vi "Set JSON Data.vi"(7 "VI Reference":refnum<vi>, 8 "error in (no error)":errorcluster, 10 "Value":string, 11 "String In":refnum<class "Cluster.lvclass">) -> (0 "error out":errorcluster, 3 "String Out":refnum<class "Cluster.lvclass">)   [LabVIEW 2017, in "Front Panel Publisher.lvlib" / "Cluster.lvclass"]
uses:
  Cluster.lvclass
  Object_class/Object.lvclass
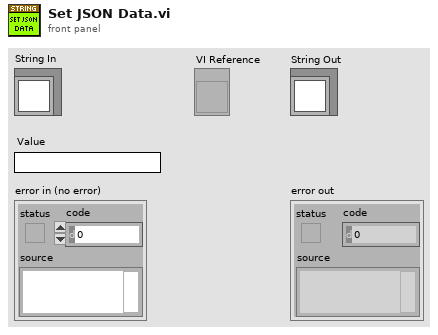
[diagram p1: front panel]
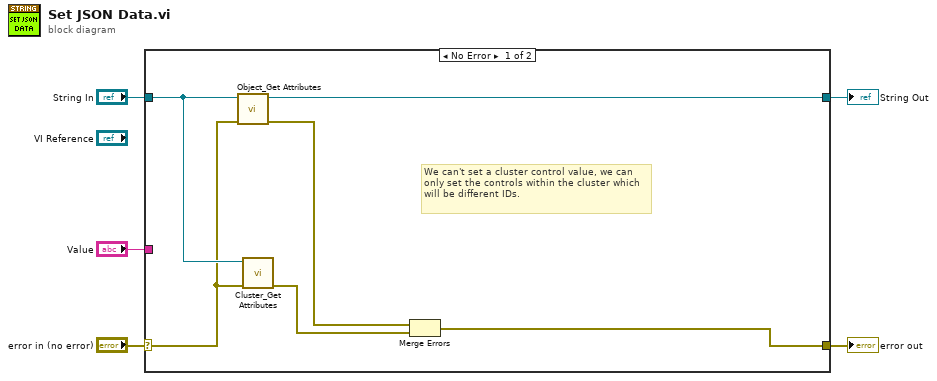
[diagram p0: block diagram]
diagram:
  n1 = case shown="No Error" "error in (no error)" {
    selector: "error in (no error)" -> [w7 w13]
    tunnel: [w6 w13] -> w4
    tunnel: [w10 w12] -> w2
    tunnel: "String In" -> [w9 w12]
    tunnel: "Value" -> [_ _]
    frame No Error {
      # "We can't set a cluster control value, we can only set the controls within the cluster which will be different IDs."
      n2 = call "Object_Get Attributes.vi"("error in (no error)"=w7, "Object In"=w9) -> ("error out"=w11:errorcluster, "Object Out"=w10:refnum<class "Cluster.lvclass">)  [unwired: 7 in, 1 out]
      n3 = call "Cluster_Get Attributes.vi"("error in (no error)"=w7, "Cluster In"=w9) -> ("error out"=w8:errorcluster)  [unwired: 7 in, 2 out]
      n4 = Merge Errors(w11, w8) -> (w6:errorcluster)
    }
    frame Error {
    }
  }
  "error out" <- w4
  "String Out" <- w2
